vi "Server Thread Handle Message.vi"   [LabVIEW 2016]
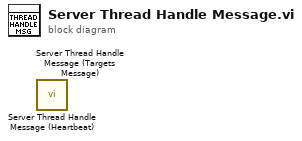
[diagram p0: block diagram]
diagram:
  n1 = call "Server Thread Handle Message (Heartbeat).vi"() -> ()  [unwired: 4 in, 3 out]
  n2 = call "Server Thread Handle Message (Targets Message).vi"() -> ()  [unwired: 4 in, 3 out]
